vi "DestroyStandardEvents.vi"(8 "error in":errorcluster, 11 "standard events":T1) -> (0 "error out":errorcluster)   [LabVIEW 2013, in "NISE_CEF_Node.lvclass"]
uses:
  NISE_CEF_Node.lvclass
  StandardEvents.ctl
  UserEventRef.ctl
  Controls/EventCluster.ctl
  NodeChangeEvent.ctl
  NodeRef.ctl
  CacheState.ctl
  RefreshUIEvent.ctl
  StopEvent.ctl
  NISE_CEF_TreeControl.lvlib
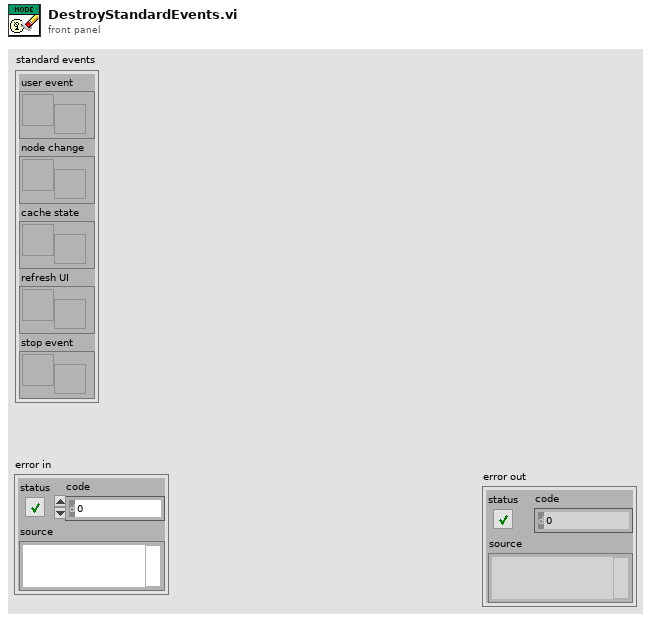
[diagram p1: front panel]
types:
  T1 = typedef "NISE_CEF_Node.lvclass/StandardEvents.ctl" = cluster{"user event":T2, "node change":T3, "cache state":T4, "refresh UI":T5, "stop event":T6}
  T2 = typedef "NISE_CEF_Node.lvclass/UserEventRef.ctl" = refnum<user-event>
  T3 = typedef "NISE_CEF_Node.lvclass/NodeChangeEvent.ctl" = refnum<user-event>
  T4 = typedef "NISE_CEF_Node.lvclass/CacheState.ctl" = refnum<user-event>
  T5 = typedef "NISE_CEF_Node.lvclass/RefreshUIEvent.ctl" = refnum<user-event>
  T6 = typedef "NISE_CEF_Node.lvclass/StopEvent.ctl" = refnum<user-event>
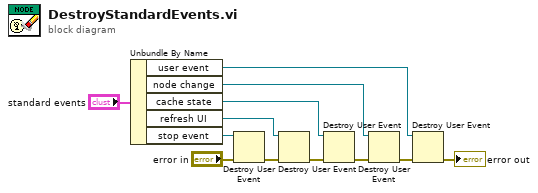
[diagram p0: block diagram]
diagram:
  n1 = Unbundle By Name("standard events") -> ("user event"=w1:T2, "node change"=w2:T3, "cache state"=w3:T4, "refresh UI"=w4:T5, "stop event"=w5:T6)
  n2 = Destroy User Event(user event=w5, error in="error in") -> (error out=w9:errorcluster)
  n3 = Destroy User Event(user event=w4, error in=w9) -> (error out=w8:errorcluster)
  n4 = Destroy User Event(user event=w3, error in=w8) -> (error out=w7:errorcluster)
  n5 = Destroy User Event(user event=w2, error in=w7) -> (error out=w6:errorcluster)
  n6 = Destroy User Event(user event=w1, error in=w6) -> (error out=→"error out":errorcluster)
